vi "Example Callback - Coordinates Callback.vi"(4 "Coordinates":refnum<user-event>, 5 "Event Data":T1, 6 "Control Ref":refnum<k24>, 7 "Event Common Data":T2) -> ()   [LabVIEW 2013]
uses:
  C:/tf/play/labview/Tinkerforge.dll
  Tinkerforge.dll
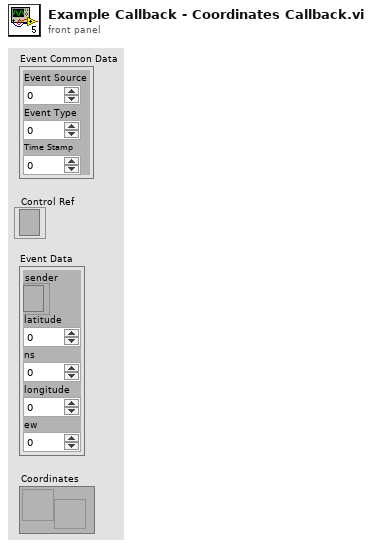
[diagram p1: front panel]
types:
  T1 = cluster{"sender":refnum<k24>, "latitude":i64, "ns":u16, "longitude":i64, "ew":u16}
  T2 = cluster{"Event Source":i32, "Event Type":u32, "Time Stamp":u32}
  T3 = cluster{"latitude":i64, "ns":u16, "longitude":i64, "ew":u16}
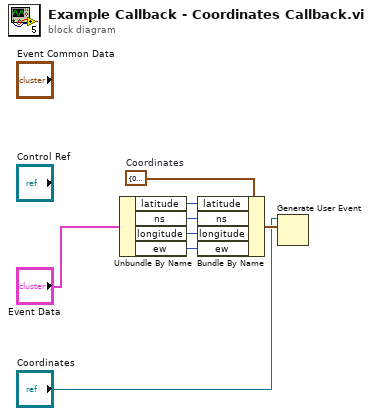
[diagram p0: block diagram]
diagram:
  w8 = T3 {"latitude"=0, "ns"=0, "longitude"=0, "ew"=0}  # Coordinates
  n1 = Unbundle By Name("Event Data") -> ("latitude"=w7:i64, "ns"=w6:u16, "longitude"=w5:i64, "ew"=w4:u16)
  n2 = Bundle By Name(cluster=w8, "latitude"=w7, "ns"=w6, "longitude"=w5, "ew"=w4) -> (w3:T3)
  n3 = Generate User Event(user event="Coordinates", event data cluster=w3) -> ()  [unwired: 2 in, 2 out]
